vi "Web Browser.vi"(1 "URL":string) -> ()   [LabVIEW 2015]
uses:
  toolbar icons/web browser back.ctl
  toolbar icons/web browser forward.ctl
panel:
  in  "Forward Button":T1
  in  "Back Button":T2
  in  "OK Button":bool
  in  "WebBrowser":refnum<k7>(container)
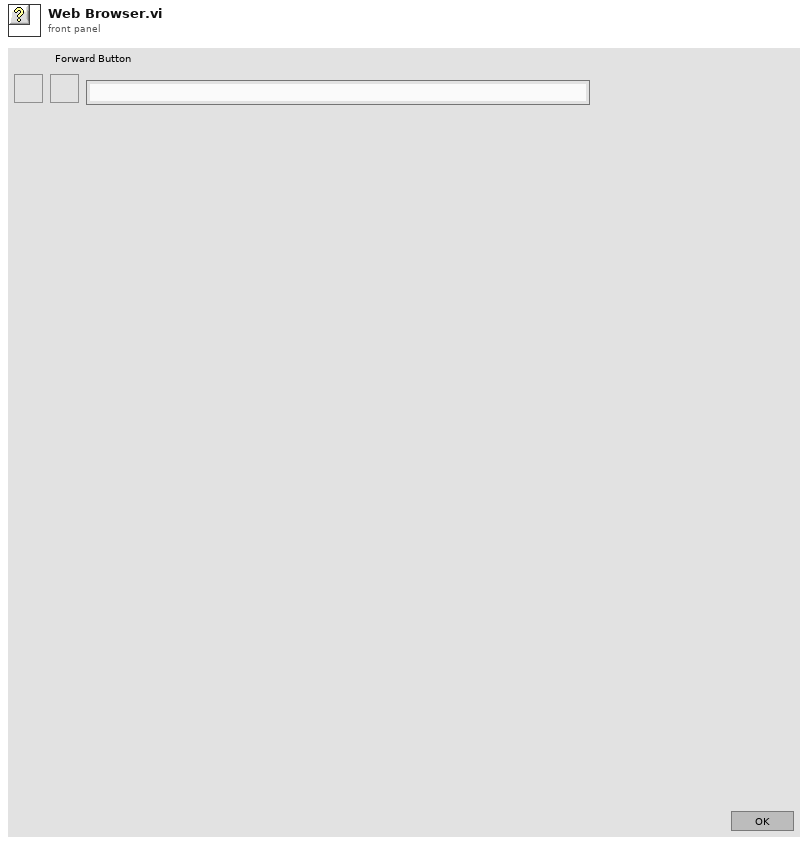
[diagram p1: front panel]
types:
  T1 = typedef "web browser forward.ctl" = bool
  T2 = typedef "web browser back.ctl" = bool
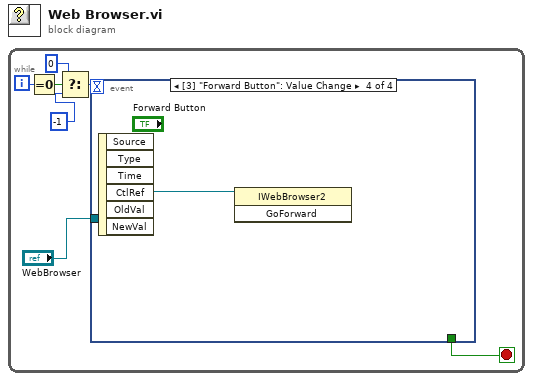
[diagram p0: block diagram]
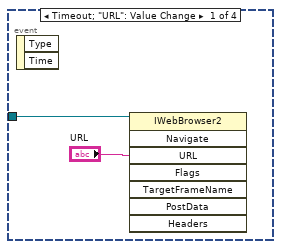
[diagram p2: hidden frame]
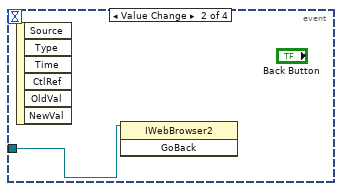
[diagram p3: hidden frame]
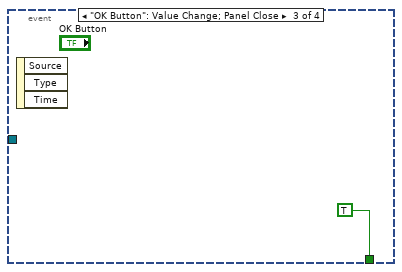
[diagram p4: hidden frame]
diagram:
  n1 = while {
    i -> [w6]
    stop <- w3 stop-if-true
    n2 = Equal To 0?(x=w6) -> (x = 0?=w7:bool)
    n3 = Select(t=0, s=w7, f=-1) -> (s? t:f=w2:i32)
    n4 = event shown="[3] \"Forward Button\": Value Change" {
      selector: _ -> [_ _ _ _]
      dyn-events: _ -> [_ _ _ _]
      timeout: w2 -> [_ _ _ _]
      tunnel: [_ _ TRUE _] -> w3
      tunnel: "WebBrowser" -> [w9 w10 _ w12]
      event Timeout; "URL": Value Change {
        n5 = event-data() -> ()  [unwired: 1 in, 2 out]
        n6 = invoke class="IWebBrowser2" method="Navigate"(reference=w9, "URL"="URL") -> ()  [unwired: 6 in, 8 out]
      }
      event Value Change {
        n7 = event-data() -> ()  [unwired: 1 in, 6 out]
        n8 = invoke class="IWebBrowser2" method="GoBack"(reference=w10) -> ()  [unwired: 2 in, 3 out]
      }
      event "OK Button": Value Change; Panel Close {
        n9 = event-data() -> ()  [unwired: 1 in, 3 out]
      }
      event Value Change {
        n10 = event-data() -> ()  [unwired: 1 in, 6 out]
        n11 = invoke class="IWebBrowser2" method="GoForward"(reference=w12) -> ()  [unwired: 2 in, 3 out]
      }
    }
  }
